vi "Plot_SkipTabbing_read.vi"(4 "error in (no error)":errorcluster, 6 "Container State":T2, 7 "Display State In":T1) -> (0 "error out":errorcluster, 2 "Value":bool, 3 "Display State Out":T1)   [LabVIEW 2018, in "XY Plot with Error Bars.xctl"]
uses:
  XY Plot with Error Bars.xctl
  <vilib>/_xctls/Container State.ctl
  State.ctl
  <vilib>/_xctls/XControlSupport.lvlib
panel:
  # "Replace the Value Indicator below with an Indicator of desired type.\nDo not remove this Indicator or the others from the connector pane. \nDo not change the connector pane pattern.\nThe Value Indicator should always be the second terminal from top on the output side in the connector pane."
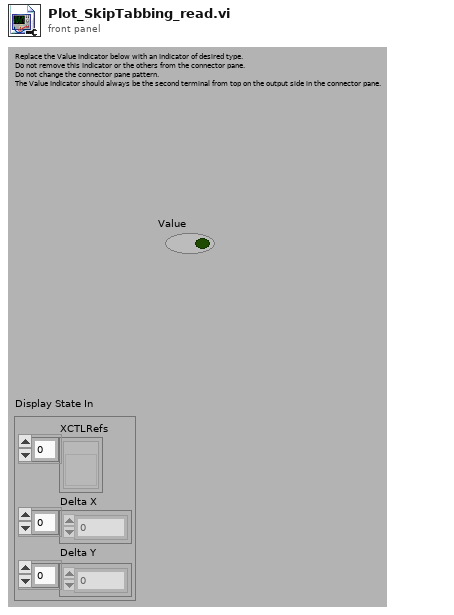
[diagram p1: front panel]
types:
  T1 = typedef "XY Plot with Error Bars.xctl/State.ctl" = cluster{"XCTLRefs":refnum<vi>[], "Delta X":dbl[], "Delta Y":dbl[]}
  T2 = typedef "XControlSupport.lvlib/Container State.ctl" = cluster{"Indicator?":bool, "Run Mode?":bool, " Refnum":refnum<vi>}
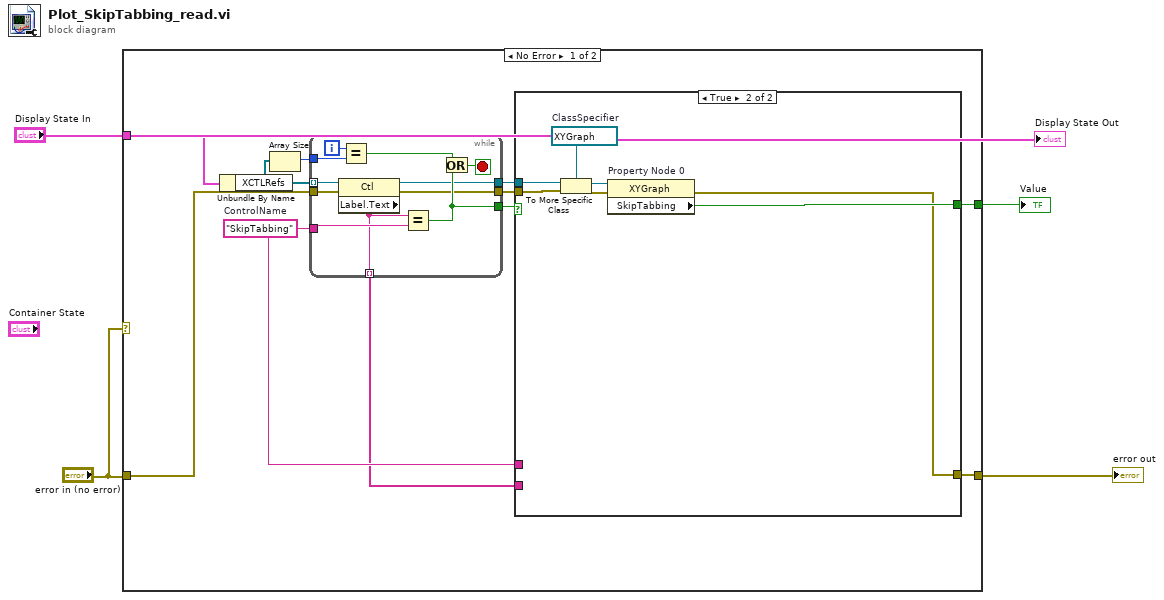
[diagram p0: block diagram]
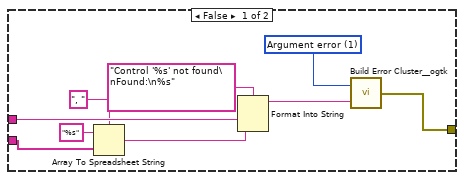
[diagram p2: hidden frame]
diagram:
  n1 = case shown="No Error" "error in (no error)" {
    tunnel: "Display State In" -> [w15 _]
    tunnel: "error in (no error)" -> [w12 w43]
    tunnel: [w9 w43] -> w2
    tunnel: [w6 _] -> w1
    frame No Error {
      w10 = "SkipTabbing"  # ControlName
      n2 = Unbundle By Name(w15) -> ("XCTLRefs"=w14:refnum<vi>[])
      n3 = Array Size(array=w14) -> (size(s)=w13:i32)
      n4 = while {
        tunnel: w14 -> [w40] mode=indexing
        tunnel: w10 -> [w38]
        tunnel: w13 -> [w41]
        tunnel: w12 -> [w39]
        tunnel: [w35] -> w11
        tunnel: [w34] -> w8
        tunnel: [w33] -> w7
        tunnel: [w32] -> w5 mode=indexing
        i -> [w42]
        stop <- w36 stop-if-true
        n5 = property class="Ctl"(reference=w40, error in=w39) -> (reference out=w34:refnum<vi>, error out=w33:errorcluster, "Label.Text"=w32:string)
        n6 = Equal?(x=w42, y=w41) -> (x = y?=w37:bool)
        n7 = Equal?(x=w32, y=w38) -> (x = y?=w35:bool)
        n8 = Or(x=w37, y=w35) -> (x .or. y?=w36:bool)
      }
      n9 = case shown="True" w11 {
        tunnel: w10 -> [w21 _]
        tunnel: [w20 w25] -> w9
        tunnel: w8 -> [_ w31]
        tunnel: w7 -> [_ w29]
        tunnel: [_ w26] -> w6
        tunnel: w5 -> [w19 _]
        frame False {
          w24 = 1 items=["No error", "Argument error", "Memory is full", "Out of zone", "End of file", "File already open", "Generic file I/O error", "File not found", "File permission error", "Disk is full", "Duplicate path", "Too many files open", "System feature not enabled", "Resource file not found", "Cannot add resource", "Resource not found", "Image not found", "Image memory error", "Pen does not exist", "Config type invalid", "Config token not found", "Config parse error", "Config memory error", "Bad external code format", "Bad external code offset", "External code not present", "Null window", "Destroy window error", "Null menu", "Print aborted", "Bad print record", "Print driver error", "Windows error during printing", "Memory error during printing", "Print dialog error", "Generic print error", "Invalid device refnum", "Device not found", "Device parameter error", "Device unit error", "Cannot open device", "Device call aborted", "Generic error", "Cancelled by user", "Object ID too low", "Object ID too high", "Object not in heap", "Unknown heap", "Unknown object (invalid DefProc)", "Unknown object (DefProc not in table)", "Message out of range", "Invalid (null) method", "Unknown message", "Manager call not supported", "Bad address", "Network operation in progress", "Network operation timed out", "Connection is busy", "Network attribute not supported", "Network error", "Address in use", "System out of memory", "Connection aborted", "Connection refused", "Not connected", "Already connected", "Connection closed", "Initialization error (interapplication manager)", "Bad occurrence", "Wait on unbound occurrence handler", "Occurrence queue overflow", "Datalog type conflict", "Unused", "Unrecognized type (interapplication manager)", "Memory corrupt", "Failed to make temporary DLL", "Old CIN version", "Drag socket not found", "Failed to load drop-object", "Failed to register OLE object", "Failed to release OLE object", "Format specifier type mismatch", "Unknown format specifier", "Too few format specifiers", "Too many format specifiers", "Scan failed", "Newer CIN version", "Error converting to variant", "Runtime menu error", "Password tampered", "Variant attribute not found", "Incompatible variant data type", "Event data is not available", "Event Store is not present", "Occurrence is not found", "Event Queue is not created", "Event info is not available", "Refnum passed is NULL", "Error retrieving Class GUID", "Error retrieving CoClass GUID", "Error retrieving TypeLib GUID.", "Bad built application magic bytes.", "Specific driver is different from the specific driver associated with the Logical Name.", "There is no session opened to the class driver.", "Max Error", "MAX - Error with config objects", "MAX - Error loading configuration", "MAX - Group not supported"]
          n10 = Array To Spreadsheet String(delimiter (Tab)=", ", array=w19, 3:"%s" ("format string")) -> (spreadsheet string=w16:string)
          n11 = Format Into String(format string="Control '%s' not found\nFound:\n%s", w21, w16) -> (resulting string=w23:string)  [unwired: 2 in, 1 out]
          n12 = call <userlib>:"Build Error Cluster__ogtk.vi"("String to Prepend to source (\"\")"=w23, "code"=w24) -> ("error out"=w20:errorcluster)
        }
        frame True {
          w30 = refnum<vi> refnum  # ClassSpecifier
          n13 = To More Specific Class(target class=w30, reference=w31, error in=w29) -> (specific class reference=w27:refnum<vi>, error out=w28:errorcluster)
          n14 = property on="Property Node 0" class="XYGraph"(reference=w27, error in=w28) -> (error out=w25:errorcluster, "SkipTabbing"=w26:bool)  [unwired: 1 out]
        }
      }
    }
    frame Error {
    }
  }
  "error out" <- w2
  "Value" <- w1
  "Display State Out" <- "Display State In"
